vi "ziTransferFunction.vi"(9 "Order (#)":i32=8, 10 "Timeconstant (s)":dbl=0.01 format="%#_3p", 11 "Frequencies (Hz)":dbl[](array[numeric])=[0.0, 1.0, 2.0, 5.0, 10.0, 40.0, 50.0, 200.0, 600.0]) -> (3 "TransferFunction":cdb[](array[numeric]))   [LabVIEW 2015, in "Zurich Instruments LabOne.lvlib"]
doc: "This vi calculates the transfer function value at the provided frequencies. The returned complex values can be used to calculate absolute values and phases. \n\nThis vi can also be used to compensate dynamic demodulated signals from filter impact both in value and phase. \n\n<B>Frequencies</B> are relative to the demodulation frequency."
uses:
  Zurich Instruments LabOne.lvlib
panel:
  out "Phase of Transfer Function":cluster{dbl[], dbl[]}(graph)
  out "Abs of Transfer Function":cluster{dbl[], dbl[]}(graph)
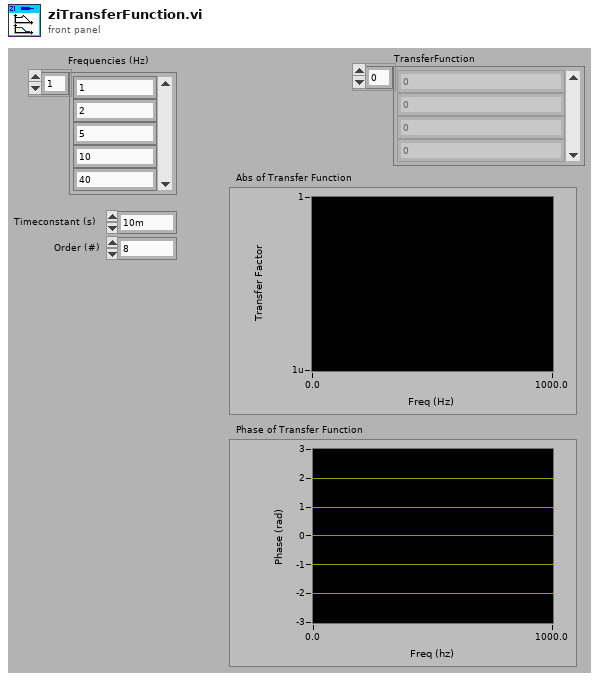
[diagram p1: front panel]
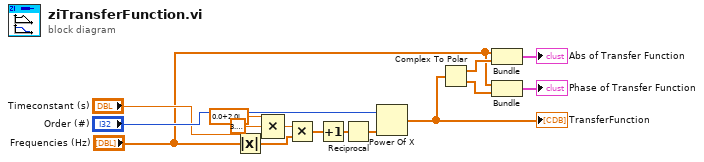
[diagram p0: block diagram]
diagram:
  n1 = Absolute Value(x="Frequencies (Hz)") -> (abs(x)=w1:dbl[])
  n2 = Compound Arithmetic op=MULTIPLY(cdb 0.0+2.0i ("r * e^(i*theta)"), 3.141592653589793, "Timeconstant (s)") -> (w5:cdb)
  n3 = Multiply(x=w5, y=w1) -> (x*y=w2:cdb[])
  n4 = Increment(x=w2) -> (x+1=w4:cdb[])
  n5 = Reciprocal(x=w4) -> (1/x=w3:cdb[])
  n6 = Power Of X(1:w3, 2:"Order (#)") -> (0:w13:cdb[])
  "TransferFunction" <- w13
  n7 = Complex To Polar(r * e^(i*theta)=w13) -> (r=w11:dbl[], theta=w9:dbl[])
  n8 = Bundle("Frequencies (Hz)"="Frequencies (Hz)", w11) -> (→"Abs of Transfer Function":cluster{"Frequencies (Hz)":dbl[], dbl[]})  [unwired: 1 in]
  n9 = Bundle("Frequencies (Hz)"="Frequencies (Hz)", w9) -> (→"Phase of Transfer Function":cluster{"Frequencies (Hz)":dbl[], dbl[]})  [unwired: 1 in]
